vi "zad2.vi"() -> ()   [LabVIEW 2017]
uses:
  Lab6/Lab6_17/Control 1.ctl
  <vilib>/sound2/lvsound2.llb/Sampling Mode.ctl
  <vilib>/sound2/lvsound2.llb/Sound Data Format.ctl
  <vilib>/measure/maspectr.llb/FFT Power Spectrum and PSD for N Chan.vi
  <vilib>/sound2/lvsound2.llb/Sound Input Read (DBL).vi
  <vilib>/measure/NI_MAPro.lvlib
panel:
  out "Power spectrum":cluster{"f0":dbl, "df":dbl, "magnitude":dbl[]}[](graph)
  in  "stop":bool
  out "error out":errorcluster
  in  "number of samples/ch 2":i32=100000
  in  "sound format":T1={"sample rate (S/s)"=22050.0, "number of channels"=2, "bits per sample"=16}
  in  "sample mode":T2=1 items=["Finite Samples", "Continuous Samples"]
  in  "device ID":u32
  out "Time Signal":waveform(dbl)[](graph)
  out "Enum":T3
  in  "?":bool
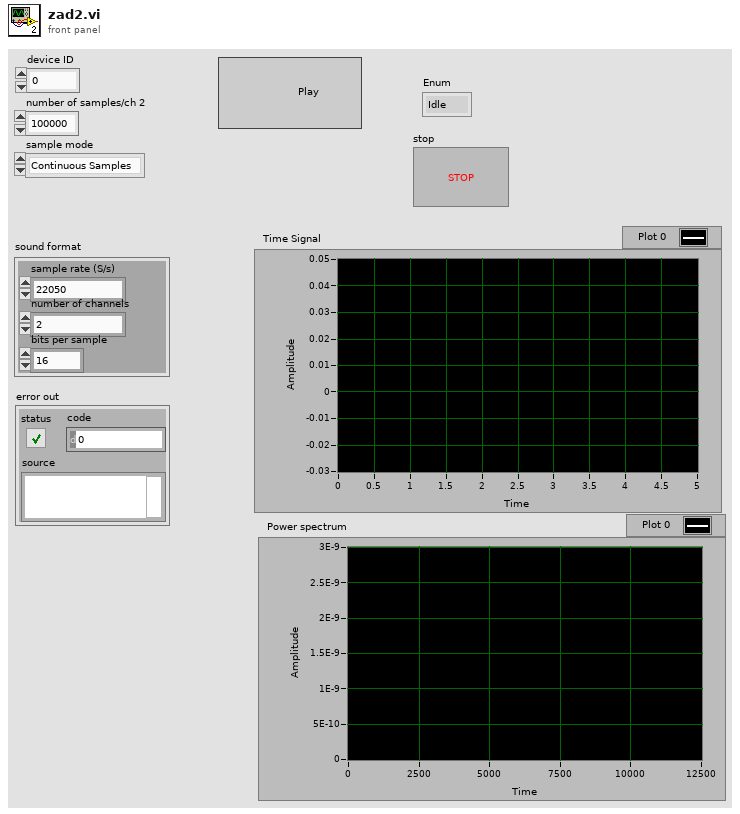
[diagram p1: front panel]
types:
  T1 = typedef "Sound Data Format.ctl" = cluster{"sample rate (S/s)":dbl, "number of channels":i32, "bits per sample":i32}
  T2 = typedef "Sampling Mode.ctl" = i32
  T3 = typedef "Control 1.ctl" = enum16{"Idle", "Initialization", "Aquisition", "End"}
  T4 = typedef "Sound Input Task ID.ctl" = u32
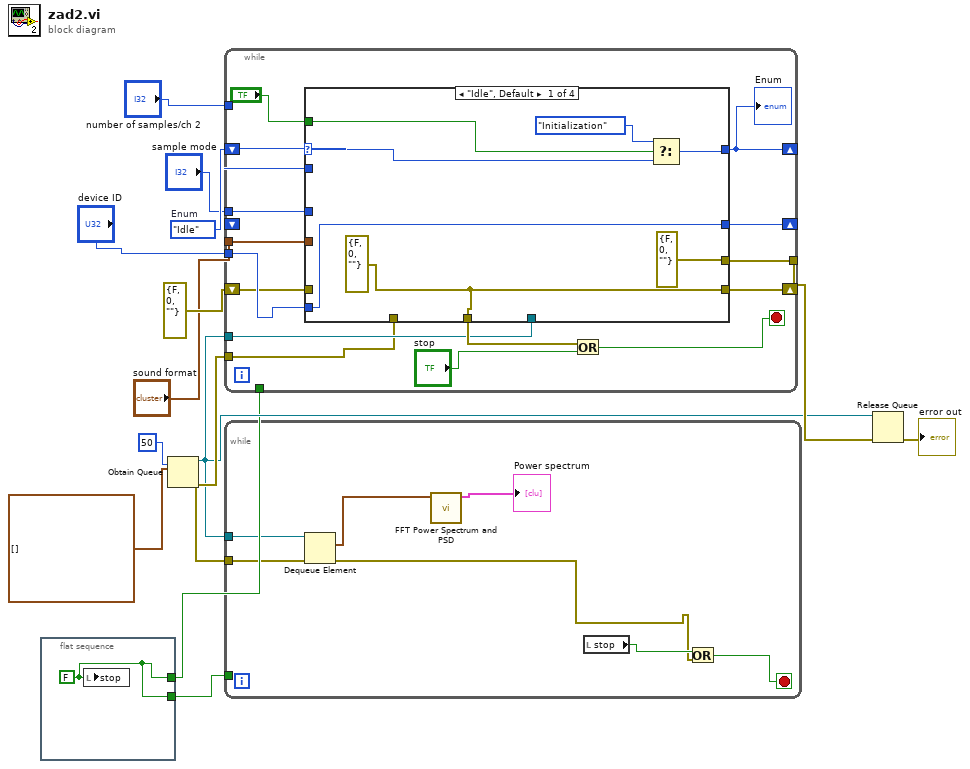
[diagram p0: block diagram]
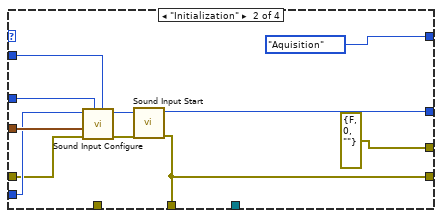
[diagram p2: hidden frame]
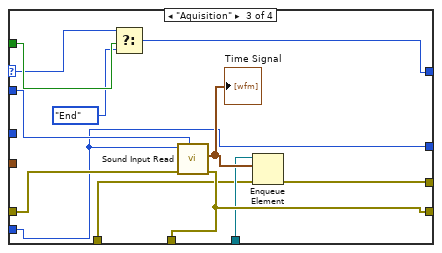
[diagram p3: hidden frame]
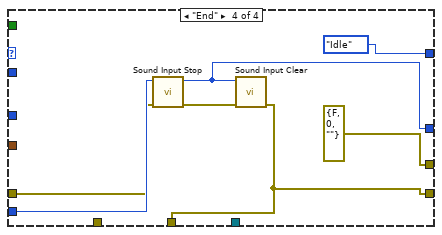
[diagram p4: hidden frame]
diagram:
  w13 = Control_1."Idle"  # Enum
  n1 = flat-sequence {
    tunnel: [w15] -> w3
    tunnel: [w15] -> w2
    frame #0 {
      w15 = FALSE ("stop")
      n2 = local write "stop"(w15) -> ()
    }
  }
  n3 = Obtain Queue(max queue size (-1, unlimited)=50, element data type=waveform(dbl)[] [] ("data")) -> (queue out=w5:refnum<queue>, error out=w7:errorcluster)  [unwired: 3 in, 1 out]
  n4 = while {
    shift-right: [w29] -> _
    shift-left: w13 -> [w25]
    shift-right: [w27] -> _
    shift-left: errorcluster {"status"=FALSE, "code"=0, "source"=""} ("error in (no error)") -> [w16]
    shift-right: [w26] -> _
    shift-left: _ -> [_]
    tunnel: "sample mode" -> [w24]
    tunnel: "sound format" -> [w23]
    tunnel: "number of samples/ch 2" -> [w22]
    tunnel: w5 -> [w21]
    tunnel: w7 -> [w20]
    tunnel: [w19] -> w6
    tunnel: "device ID" -> [w17]
    tunnel: w3 -> [_]
    stop <- w30 stop-if-true
    n5 = case shown="\"Idle\", Default" w25 {
      selector: w25 -> [w35 _ w56 _]
      tunnel: [w37 Control_1."Aquisition" ("Enum") w58 Control_1."Idle" ("Enum")] -> w29
      tunnel: "?" -> [w38 _ w60 _]
      tunnel: [w34 w49 w61 w66] -> w31
      tunnel: [w34 w49 w61 w66] -> w27
      tunnel: [w33 w48 w50 w67] -> w26
      tunnel: w23 -> [_ w44 _ _]
      tunnel: w24 -> [_ w43 _ _]
      tunnel: w22 -> [_ w42 w57 _]
      tunnel: w17 -> [w33 w41 w50 w64]
      tunnel: w21 -> [_ _ w54 _]
      tunnel: w20 -> [_ _ w53 _]
      tunnel: [errorcluster {"status"=FALSE, "code"=0, "source"=""} ("error in (no error)") errorcluster {"status"=FALSE, "code"=0, "source"=""} ("error in (no error)") w52 errorcluster {"status"=FALSE, "code"=0, "source"=""} ("error in (no error)")] -> w19
      tunnel: w16 -> [_ w39 w51 w62]
      frame "Idle", Default {
        w34 = errorcluster {"status"=FALSE, "code"=0, "source"=""} ("error out")
        n6 = Select(t=Control_1."Initialization" ("Enum"), s=w38, f=w35) -> (s? t:f=w37:T3)
      }
      frame "Initialization" {
        n7 = call <vilib>:"Sound Input Configure.vi"("number of samples/ch"=w42, "sample mode"=w43, "error in (no error)"=w39, "sound format"=w44, "device ID"=w41) -> ("error out"=w45:errorcluster, "task ID"=w46:T4)  [unwired: 5 in]
        n8 = call <vilib>:"Sound Input Start.vi"("error in (no error)"=w45, "task ID"=w46) -> ("error out"=w49:errorcluster, "task ID out"=w48:T4)  [unwired: 8 in]
      }
      frame "Aquisition" {
        n9 = Select(t=w56, s=w60, f=Control_1."End" ("Enum")) -> (s? t:f=w58:T3)
        n10 = call-poly <vilib>:"Sound Input Read.vi"("number of samples/ch"=w57, "error in (no error)"=w51, "task ID"=w50) -> ("error out"=w61:errorcluster, "data"=w55:waveform(dbl)[])  [unwired: 6 in, 1 out]
        "Time Signal" <- w55
        n11 = Enqueue Element(queue=w54, element=w55, error in (no error)=w53) -> (error out=w52:errorcluster)  [unwired: 1 in, 2 out]
      }
      frame "End" {
        n12 = call <vilib>:"Sound Input Stop.vi"("error in (no error)"=w62, "task ID"=w64) -> ("error out"=w68:errorcluster, "task ID out"=w67:T4)  [unwired: 8 in]
        n13 = call <vilib>:"Sound Input Clear.vi"("error in (no error)"=w68, "task ID"=w67) -> ("error out"=w66:errorcluster)  [unwired: 9 in]
      }
    }
    "Enum" <- w29
    n14 = Or(x=w31, y="stop") -> (x .or. y?=w30:bool)
  }
  n15 = while {
    tunnel: w5 -> [w75]
    tunnel: w7 -> [w74]
    tunnel: w2 -> [_]
    stop <- w69 stop-if-true
    n16 = Dequeue Element(queue=w75, error in (no error)=w74) -> (element=w73:waveform(dbl)[], error out=w70:errorcluster)  [unwired: 1 in, 2 out]
    n17 = call-poly <vilib>:"FFT Power Spectrum and PSD.vi"("time signals"=w73) -> ("Power Spectrum / PSD"=→"Power spectrum":cluster{"f0":dbl, "df":dbl, "magnitude":dbl[]}[])  [unwired: 7 in, 3 out]
    n18 = local read "stop"() -> (w71:bool)
    n19 = Or(x=w71, y=w70) -> (x .or. y?=w69:bool)
  }
  n20 = Release Queue(queue=w5, error in (no error)=w6) -> (error out=→"error out":errorcluster)  [unwired: 1 in, 2 out]
